vi "Obtain Session.vi"(0 "Options":T1, 2 "Engine":T2, 11 "error in (no error)":errorcluster) -> (4 "Session Handle":T3, 15 "error out":errorcluster)   [LabVIEW 2020, in "TSS.lvlib" / "Execution.lvclass"]
doc: "This function initializes the measurement\n\nPass the function a name to obtain an active measurement handle"
uses:
  Execution.lvclass
  Typedefs/Session Handle.ctl
  C:/Program Files (x86)/National Instruments/LabVIEW 2020/user.lib/_Session Fwk/Session - Root.lvclass
  Engine/Typedefs/Session Handle.ctl
  Engine/Engine.lvclass
  Execution Options.ctl
  Execution.lvclass/Execution.ctl
  <userlib>/_Session Fwk/Session - Root.lvclass
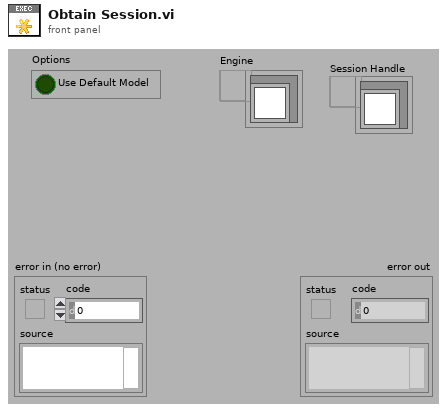
[diagram p1: front panel]
types:
  T1 = typedef "TSS.lvlib/Execution.lvclass/Execution Options.ctl" = cluster{"Use Default Model":bool}
  T2 = typedef "TSS.lvlib/Engine.lvclass/Session Handle.ctl" = refnum<data-value>
  T3 = typedef "TSS.lvlib/Execution.lvclass/Session Handle.ctl" = refnum<data-value>
  T4 = typedef "Session - Root.lvclass/Session Handle.ctl" = refnum<data-value>
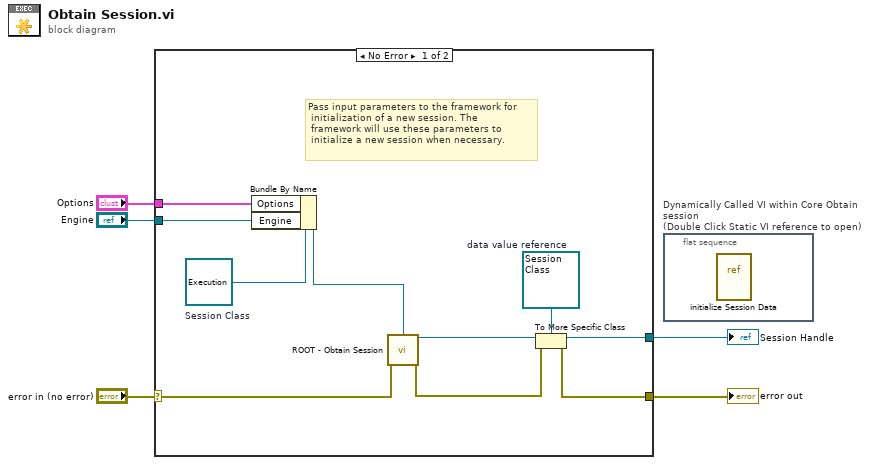
[diagram p0: block diagram]
diagram:
  n1 = case shown="No Error" "error in (no error)" {
    selector: "error in (no error)" -> [w15 w16]
    tunnel: [w12 w16] -> w4
    tunnel: [w14 _] -> w3
    tunnel: "Engine" -> [w9 _]
    tunnel: "Options" -> [w6 _]
    frame No Error {
      w7 = refnum<data-value> refnum  # data value reference
      w8 = refnum<class "Execution.lvclass"> refnum  # Session Class
      # "Pass input parameters to the framework for\n initialization of a new session. The\n framework will use these parameters to\n initialize a new session when necessary."
      n2 = Bundle By Name(cluster=w8, "Options"=w6, "Engine"=w9) -> (w10:refnum<class "Execution.lvclass">)
      n3 = call <userlib>:"ROOT - Obtain Session.vi"("OBJ - Session"=w10, "error in (no error)"=w15) -> ("Session Handle"=w11:T4, "error out"=w13:errorcluster)  [unwired: 11 in, 1 out]
      n4 = To More Specific Class(target class=w7, reference=w11, error in=w13) -> (specific class reference=w14:refnum<data-value>, error out=w12:errorcluster)
    }
    frame Error {
    }
  }
  "error out" <- w4
  "Session Handle" <- w3
  n5 = flat-sequence "Dynamically Called VI within Core Obtain session\n(Double Click Static VI reference to open)" {
    frame #0 {
      n6 = vi-ref "initialize Session Data.vi"() -> ()  [unwired: 1 out]
    }
  }
